vi "Default Events--constant.vi"() -> (3 "Default Event Names":string[](array[string]))   [LabVIEW 2021, in "TAF Proj Document Type.lvlib" / "Dqmh Module.lvclass"]
uses:
  <vilib>/Wovalab/AntiDoc/Document Type/Add-ons/LabVIEW TAF Project/Dqmh Module/Dqmh Module.lvclass
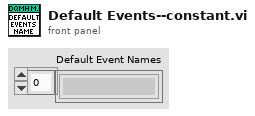
[diagram p1: front panel]
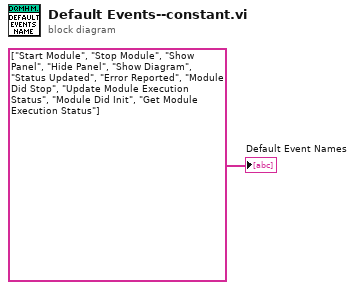
[diagram p0: block diagram]
diagram:
  "Default Event Names" <- string[] ["Start Module", "Stop Module", "Show Panel", "Hide Panel", "Show Diagram", "Status Updated", "Error Reported", "Module Did Stop", "Update Module Execution Status", "Module Did Init", "Get Module Execution Status"] ("Default Event Names")
